vi "QCA Pick Baseline.vi"(1 "QMeter":string, 2 "Current Baseline":i32) -> (0 "New Baseline":i32)   [LabVIEW 2010]
doc: "This VI is called by the QCA. Its purpose is to present the user with a range of choices for what baseline to use. The user can pick from existing baselines for the current Q Meter, or can opt to take a new baseline."
uses:
  TCL-Target_Computer_Logging/TCL Select Base Fragments/TCL Select Base Fragments NfragsNcriteria.vi
panel:
  in  "No Baseline":bool
  in  "Cancel":bool
  in  "New Baseline":bool
  in  "Choose Baseline":bool
  out "Raw Signal of Highlighted Baseline":dbl[](graph)
  in  "To choose an existing baseline, select from this list":i32(listbox)
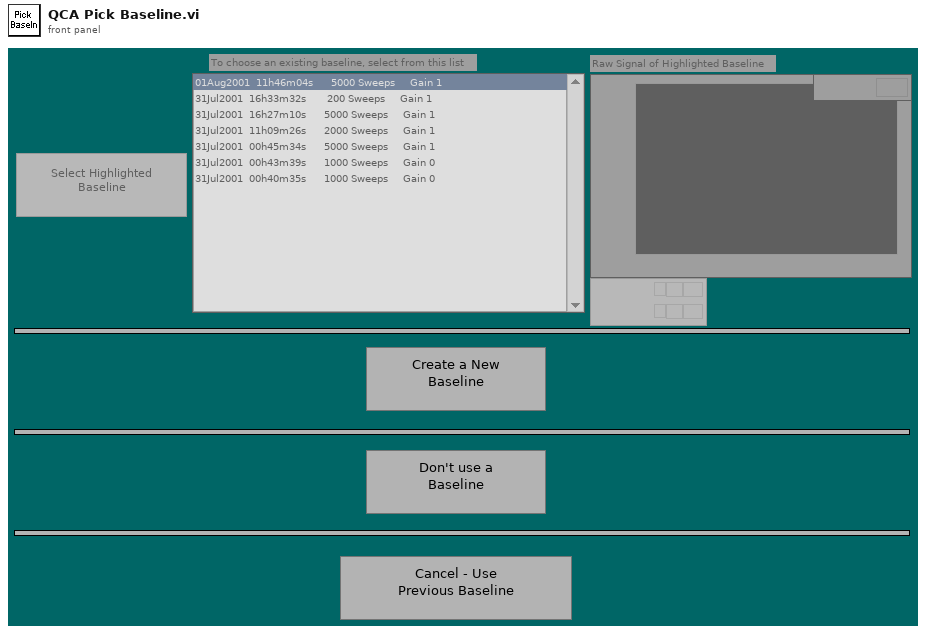
[diagram p1: front panel]
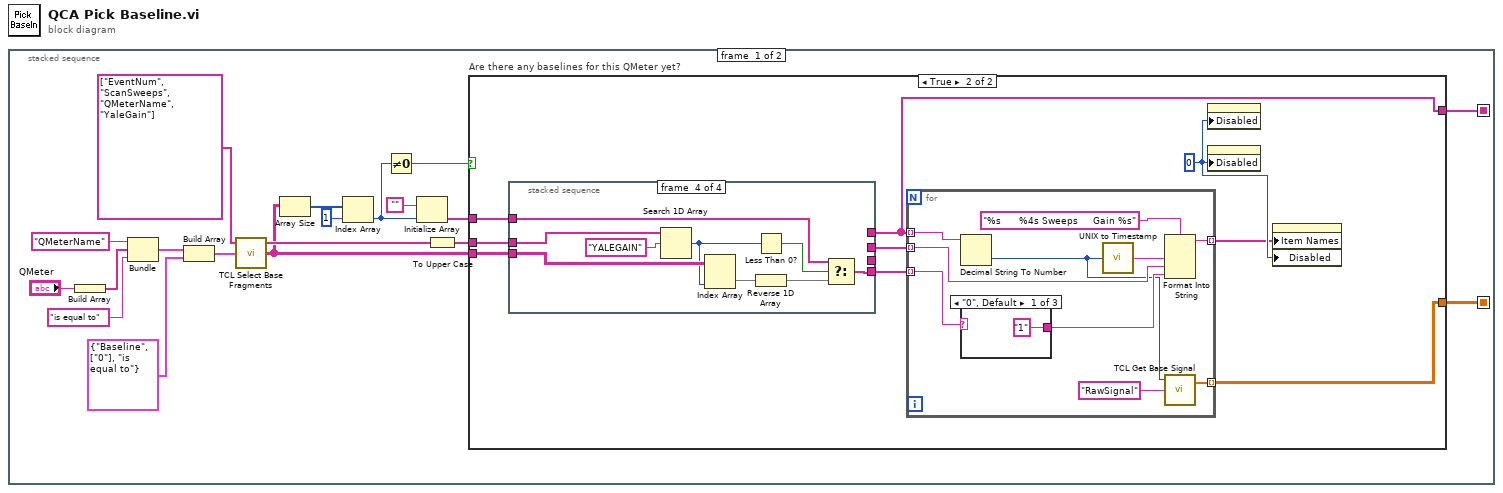
[diagram p0: block diagram]
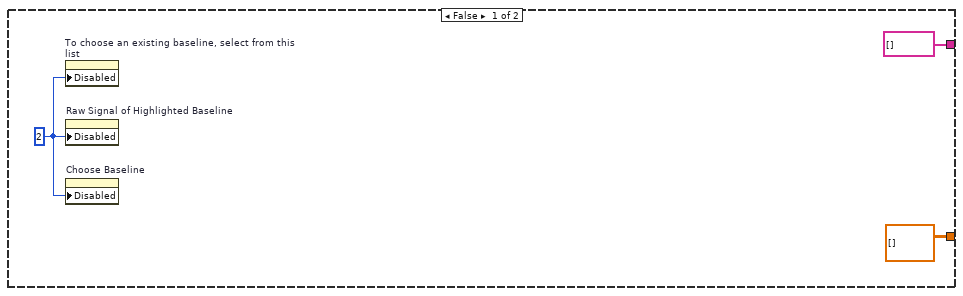
[diagram p2: hidden frame]
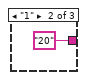
[diagram p3: hidden frame]
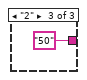
[diagram p4: hidden frame]
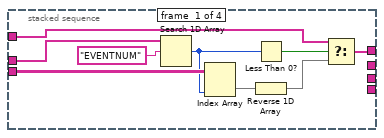
[diagram p5: hidden frame]
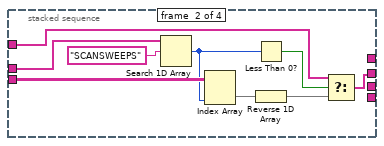
[diagram p6: hidden frame]
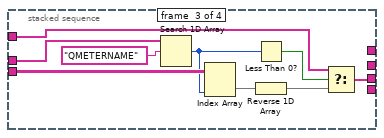
[diagram p7: hidden frame]
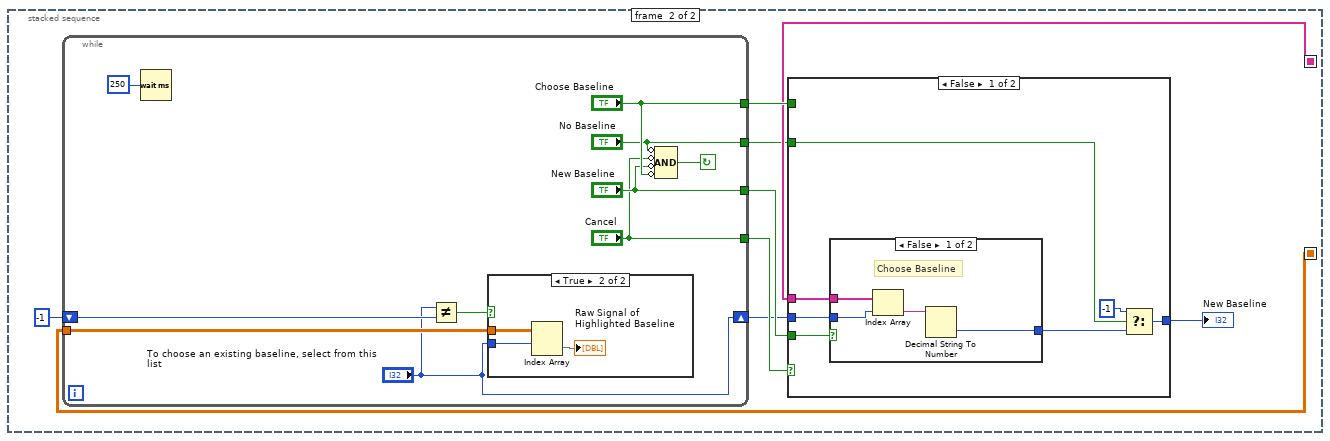
[diagram p8: hidden frame]
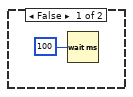
[diagram p9: hidden frame]
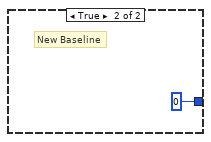
[diagram p10: hidden frame]
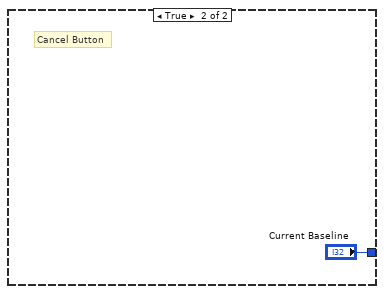
[diagram p11: hidden frame]
diagram:
  n1 = stacked-sequence {
    seq-local: [w8 _] -> [_ w88]
    seq-local: [w7 _] -> [_ w83]
    frame #0 {
      n2 = Build Array("QMeter") -> (w17:string[])
      n3 = Bundle("QMeterName", w17, "is equal to") -> (w16:cluster{string, string[], string})  [unwired: 1 in]
      n4 = Build Array(w16, cluster{string, string[], string} {"Baseline", ["0"], "is equal to"}) -> (w14:cluster{string, string[], string}[])
      n5 = call-poly "TCL Select Base Fragments .vi"("criteria"=w14, "fragments"=string[] ["EventNum", "ScanSweeps", "QMeterName", "YaleGain"]) -> ("matches"=w10:string[][], "fragments out"=w11:string[])  [unwired: 1 in, 1 out]
      n6 = Array Size(array=w10) -> (size(s)=w6:i32[])
      n7 = Index Array(array=w6, index=1) -> (element=w4:i32)
      n8 = Not Equal To 0?(x=w4) -> (x != 0?=w12:bool)
      n9 = Initialize Array("", w4) -> (w2:string[])
      n10 = To Upper Case(1:w11) -> (0:w9:string[])
      n11 = case "Are there any baselines for this QMeter yet?" shown="True" w12 {
        tunnel: w9 -> [_ w31]
        tunnel: w10 -> [_ w30]
        tunnel: [dbl[][] [] ("Raw Signal") w25] -> w8
        tunnel: [string[] [] ("Event Data") w26] -> w7
        tunnel: w2 -> [_ w27]
        frame False {
          w22 = 2
          n12 = property on="To choose an existing baseline, select from this list" class="LstBox (strict)"("Disabled"=w22) -> ()  [unwired: 2 in, 2 out]
          n13 = property on="Raw Signal of Highlighted Baseline" class="WFGraph (strict)"("Disabled"=w22) -> ()  [unwired: 2 in, 2 out]
          n14 = property on="Choose Baseline" class="Bool"("Disabled"=w22) -> ()  [unwired: 2 in, 2 out]
        }
        frame True {
          w28 = u8 0
          n15 = stacked-sequence {
            tunnel: w30 -> [w52 w61 w70 w79]
            tunnel: w31 -> [w51 w60 w69 w78]
            tunnel: [w46 _ _ _] -> w26
            tunnel: [_ w55 _ _] -> w29
            tunnel: [_ _ w64 _] -> _
            tunnel: w27 -> [w50 w59 w68 w77]
            tunnel: [_ _ _ w73] -> w23
            frame #0 {
              n16 = Search 1D Array(1D array=w51, element="EVENTNUM") -> (index of element=w47:i32)  [unwired: 1 in]
              n17 = Index Array(array=w52, index (col)=w47) -> (element=w49:string[])  [unwired: 1 in]
              n18 = Less Than 0?(x=w47) -> (x < 0?=w48:bool)
              n19 = Reverse 1D Array(array=w49) -> (reversed array=w45:string[])
              n20 = Select(t=w50, s=w48, f=w45) -> (s? t:f=w46:string[])
            }
            frame #1 {
              n21 = Search 1D Array(1D array=w60, element="SCANSWEEPS") -> (index of element=w56:i32)  [unwired: 1 in]
              n22 = Index Array(array=w61, index (col)=w56) -> (element=w58:string[])  [unwired: 1 in]
              n23 = Less Than 0?(x=w56) -> (x < 0?=w57:bool)
              n24 = Reverse 1D Array(array=w58) -> (reversed array=w54:string[])
              n25 = Select(t=w59, s=w57, f=w54) -> (s? t:f=w55:string[])
            }
            frame #2 {
              n26 = Search 1D Array(1D array=w69, element="QMETERNAME") -> (index of element=w65:i32)  [unwired: 1 in]
              n27 = Index Array(array=w70, index (col)=w65) -> (element=w67:string[])  [unwired: 1 in]
              n28 = Less Than 0?(x=w65) -> (x < 0?=w66:bool)
              n29 = Reverse 1D Array(array=w67) -> (reversed array=w63:string[])
              n30 = Select(t=w68, s=w66, f=w63) -> (s? t:f=w64:string[])
            }
            frame #3 {
              n31 = Search 1D Array(1D array=w78, element="YALEGAIN") -> (index of element=w74:i32)  [unwired: 1 in]
              n32 = Index Array(array=w79, index (col)=w74) -> (element=w76:string[])  [unwired: 1 in]
              n33 = Less Than 0?(x=w74) -> (x < 0?=w75:bool)
              n34 = Reverse 1D Array(array=w76) -> (reversed array=w72:string[])
              n35 = Select(t=w77, s=w75, f=w72) -> (s? t:f=w73:string[])
            }
          }
          n36 = for {
            tunnel: w26 -> [w41] mode=indexing
            tunnel: w29 -> [w37] mode=indexing
            tunnel: w23 -> [w36] mode=indexing
            tunnel: [w38] -> w24 mode=indexing
            tunnel: [w34] -> w25 mode=indexing
            n37 = Decimal String To Number(string=w41) -> (number=w33:i32)  [unwired: 2 in, 1 out]
            n38 = case shown="\"0\", Default" w36 {
              tunnel: ["1" "20" "50"] -> w35
              frame "0", Default {
              }
              frame "1" {
              }
              frame "2" {
              }
            }
            n39 = call "UNIX to Timestamp.vi"("Seconds"=w33) -> ("Timestamp String"=w40:string)
            n40 = Format Into String(format string="%s      %4s Sweeps     Gain %s", w40, w37, w35) -> (resulting string=w38:string)  [unwired: 2 in, 1 out]
            n41 = call "TCL Get Base Signal.vi"("signal name"="RawSignal", "event number"=w33) -> ("signal"=w34:dbl[])  [unwired: 1 in, 1 out]
          }
          n42 = property on="Raw Signal of Highlighted Baseline" class="WFGraph (strict)"("Disabled"=w28) -> ()  [unwired: 2 in, 2 out]
          n43 = property on="Choose Baseline" class="Bool"("Disabled"=w28) -> ()  [unwired: 2 in, 2 out]
          n44 = property on="To choose an existing baseline, select from this list" class="LstBox (strict)"("Item Names"=w24, "Disabled"=w28) -> ()  [unwired: 2 in, 2 out]
        }
      }
    }
    frame #1 {
      n45 = while {
        tunnel: ["No Baseline"] -> w81
        tunnel: ["Cancel"] -> w87
        tunnel: ["New Baseline"] -> w86
        tunnel: ["Choose Baseline"] -> w85
        tunnel: w88 -> [w97]
        shift-left: -1 -> [w99]
        shift-right: ["To choose an existing baseline, select from this list"] -> w84
        stop <- w95 continue-if-true
        n46 = Wait (ms)(milliseconds to wait=u32 250) -> ()  [unwired: 1 out]
        n47 = Not Equal?(x="To choose an existing baseline, select from this list", y=w99) -> (x != y?=w98:bool)
        n48 = case shown="True" w98 {
          tunnel: w97 -> [_ w102]
          tunnel: "To choose an existing baseline, select from this list" -> [_ w103]
          frame False {
            n49 = Wait (ms)(milliseconds to wait=u32 100) -> ()  [unwired: 1 out]
          }
          frame True {
            n50 = Index Array(array=w102, index (row)=w103) -> (element=→"Raw Signal of Highlighted Baseline":dbl[])  [unwired: 1 in]
          }
        }
        n51 = Compound Arithmetic op=AND(invert "No Baseline", invert "Cancel", invert "New Baseline", invert "Choose Baseline") -> (w95:bool)
      }
      n52 = case shown="False" w87 {
        tunnel: w86 -> [w108 _]
        tunnel: w85 -> [_ _]
        tunnel: [w107 "Current Baseline"] -> w82
        tunnel: w84 -> [w110 _]
        tunnel: w83 -> [w109 _]
        tunnel: w81 -> [w105 _]
        frame False {
          n53 = case shown="False" w108 {
            tunnel: [w111 0] -> w106
            tunnel: w110 -> [w114 _]
            tunnel: w109 -> [w113 _]
            frame False {
              # "Choose Baseline"
              n54 = Index Array(array=w113, index=w114) -> (element=w112:string)
              n55 = Decimal String To Number(string=w112) -> (number=w111:i32)  [unwired: 2 in, 1 out]
            }
            frame True {
              # "New Baseline"
            }
          }
          n56 = Select(t=-1, s=w105, f=w106) -> (s? t:f=w107:i32)
        }
        frame True {
          # "Cancel Button"
        }
      }
      "New Baseline" <- w82
    }
  }
